vi "Event Log.Record Status Message and Even.vi"(6 "Status Color(Lt Grey)":u32(colorbox)=13816530, 7 "Log Level(Normal)":T1, 8 "error in (no error)":errorcluster, 9 "Status Msg":string, 10 "Event Log":string, 11 "Status":T2) -> (0 "error out":errorcluster)   [LabVIEW 2024, in "EQMF.lvlib" / "Event Log.lvlib"]
uses:
  Event Log.lvlib
  Event Log.Log Params.ctl
  Event Notification/Event Log.Log Level.ctl
  Queues/Q.Element.ctl
  Queues/Queue Utils.lvlib
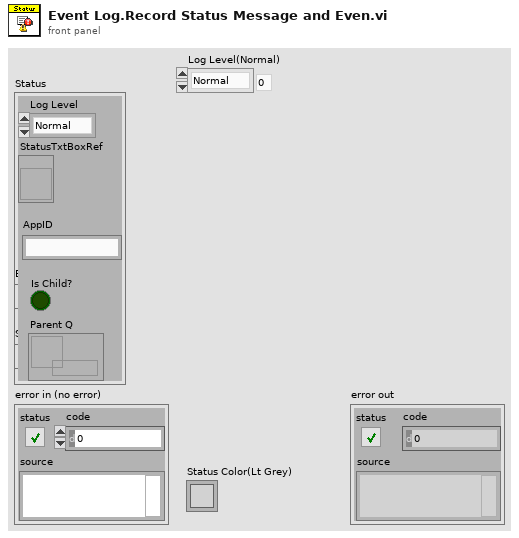
[diagram p1: front panel]
types:
  T1 = typedef "EQMF.lvlib/Event Log.lvlib/Event Log.Log Level.ctl" = enum16{"Normal", "Verbose", "Debug0", "Debug1", "Debug2"}
  T2 = typedef "EQMF.lvlib/Event Log.lvlib/Event Log.Log Params.ctl" = cluster{"Log Level":T1, "StatusTxtBoxRef":refnum<vi>, "AppID":string, "Is Child?":bool, "Parent Q":refnum<queue>}
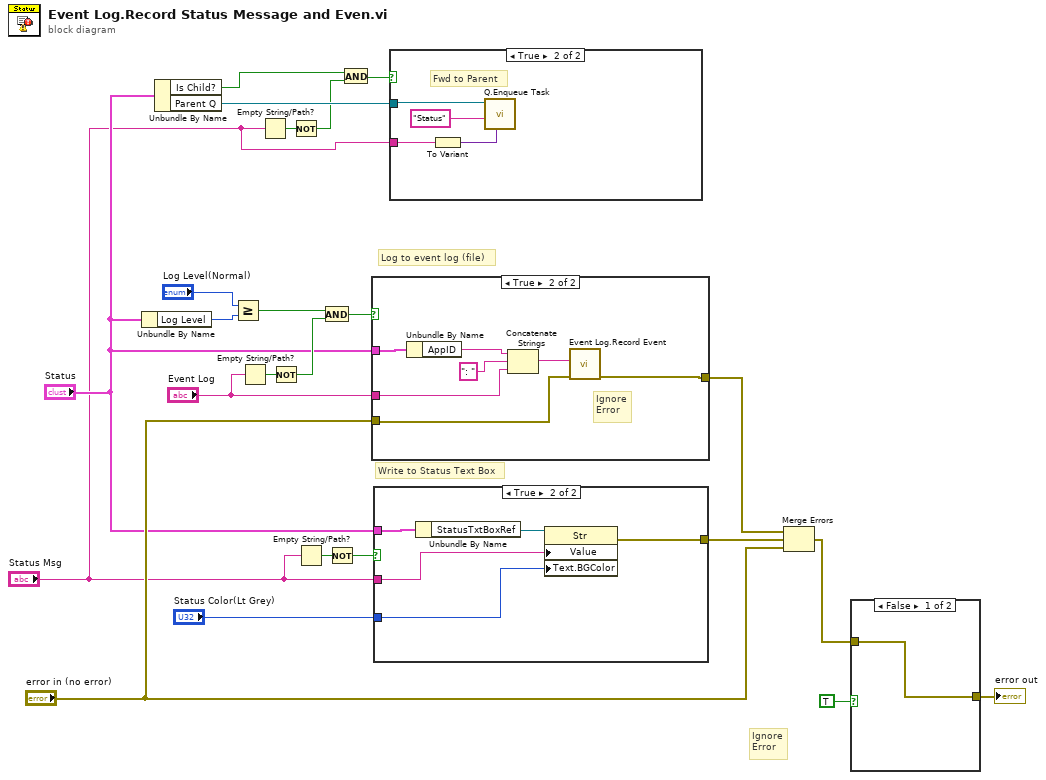
[diagram p0: block diagram]
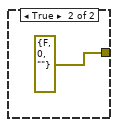
[diagram p2: hidden frame]
diagram:
  # "Ignore\nError"
  # "Write to Status Text Box"
  # "Log to event log (file)"
  n1 = Unbundle By Name("Status") -> ("Log Level"=w22:T1)
  n2 = Unbundle By Name("Status") -> ("Is Child?"=w6:bool, "Parent Q"=w9:refnum<queue>)
  n3 = Greater Or Equal?(x="Log Level(Normal)", y=w22) -> (x >= y?=w20:bool)
  n4 = Empty String/Path?(string/path="Event Log") -> (empty?=w18:bool)
  n5 = Empty String/Path?(string/path="Status Msg") -> (empty?=w8:bool)
  n6 = Not(x=w18) -> (.not. x?=w17:bool)
  n7 = Not(x=w8) -> (.not. x?=w5:bool)
  n8 = Empty String/Path?(string/path="Status Msg") -> (empty?=w15:bool)
  n9 = And(x=w20, y=w17) -> (x .and. y?=w21:bool)
  n10 = Not(x=w15) -> (.not. x?=w14:bool)
  n11 = And(x=w6, y=w5) -> (x .and. y?=w7:bool)
  n12 = case shown="True" w21 {
    tunnel: "Event Log" -> [_ w27]
    tunnel: "Status" -> [_ w30]
    tunnel: [_ w25] -> w13
    tunnel: "error in (no error)" -> [_ w24]
    frame False {
    }
    frame True {
      # "Ignore\nError"
      n13 = Unbundle By Name(w30) -> ("AppID"=w29:string)
      n14 = Concatenate Strings(w29, ": ", w27) -> (w26:string)
      n15 = call "Event Log.Record Event.vi"("error in"=w24, "Message"=w26) -> ("error out"=w25:errorcluster)  [unwired: 9 in]
    }
  }
  n16 = case shown="True" w14 {
    tunnel: "Status" -> [_ w35]
    tunnel: "Status Color(Lt Grey)" -> [_ w33]
    tunnel: "Status Msg" -> [_ w32]
    tunnel: [_ w31] -> w12
    frame False {
    }
    frame True {
      n17 = Unbundle By Name(w35) -> ("StatusTxtBoxRef"=w34:refnum<vi>)
      n18 = property class="Str"(reference=w34, "Value"=w32, "Text.BGColor"=w33) -> (error out=w31:errorcluster)  [unwired: 1 in, 1 out]
    }
  }
  n19 = case shown="True" w7 {
    tunnel: w9 -> [_ w39]
    tunnel: "Status Msg" -> [_ w36]
    frame False {
    }
    frame True {
      # "Fwd to Parent"
      n20 = To Variant(anything=w36) -> (Variant=w37:variant)
      n21 = call "Q.Enqueue Task.vi"("Data1"=w37, "Task Name"="Status", "Q In"=w39) -> ()  [unwired: 7 in, 2 out]
    }
  }
  n22 = Merge Errors(w13, w12, "error in (no error)") -> (w1:errorcluster)
  n23 = case shown="False" TRUE {
    tunnel: [w40 errorcluster {"status"=FALSE, "code"=0, "source"=""} ("error constant")] -> w2
    tunnel: w1 -> [w40 _]
    frame False {
    }
    frame True {
    }
  }
  "error out" <- w2
